vi "Thermal_Camera_Stream.vi"() -> ()   [LabVIEW 2024]
uses:
  <vilib>/userDefined/High Color/IMAQdx.ctl
  <vilib>/vision/driver/NI_Vision_Acquisition_Software.lvlib
panel:
  out "Error Config":errorcluster
  out "error Open":errorcluster
  in  "save":bool
  out "FocusPos":u32
  in  "Scale":u32=13
  in  "Focus >":bool
  in  "Focus <":bool
  in  "Focus":bool
  in  "Numeric":u16
  in  "path":string
  out "error out":errorcluster
  in  "Stop":bool
  in  "Session In":T1="cam4"
  out "Image":T2(plugin-control)
  out "Intensity Graph 2":dbl[][](graph)
  out "Temperature":dbl
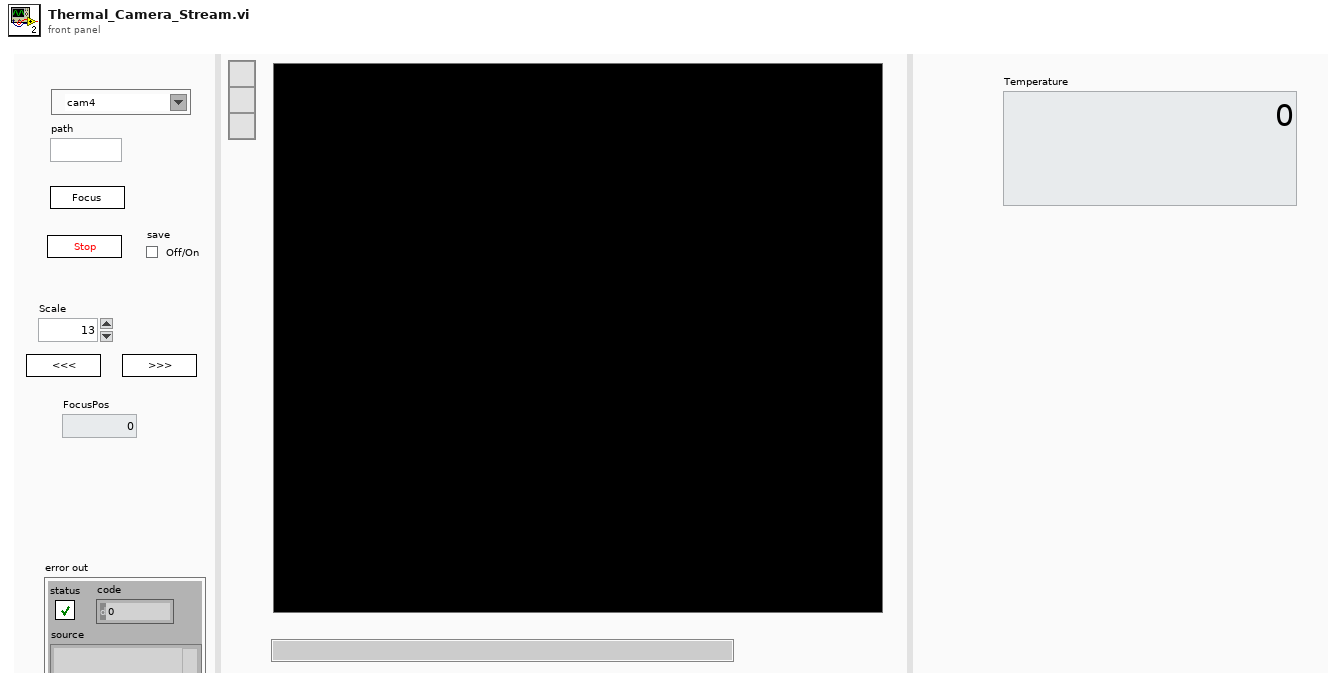
[diagram p1: front panel]
types:
  T1 = typedef "IMAQdx.ctl" = refnum<k21>
  T2 = typedef "IMAQ Image.ctl" = refnum<image>
  T3 = typedef "Image Type" = u32
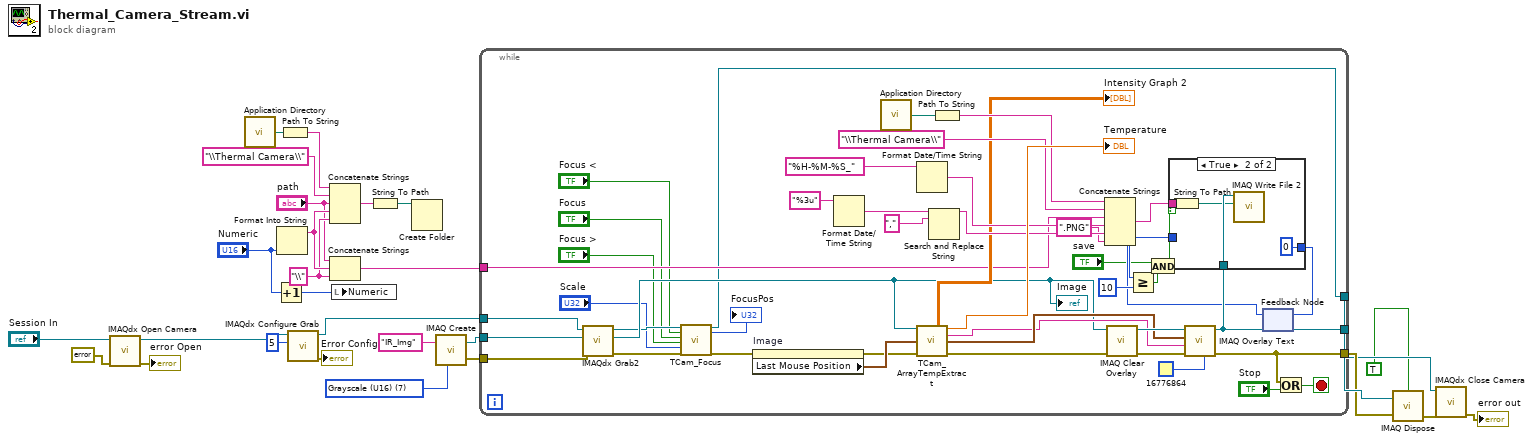
[diagram p0: block diagram]
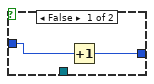
[diagram p2: hidden frame]
diagram:
  w6 = "\\" ("string")
  w17 = T3 7 items=["Grayscale (U8)", "Grayscale (I16)", "Grayscale (SGL)", "Complex (CSG)", "RGB (U32)", "HSL (U32)", "RGB (U64)", "Grayscale (U16)"] ("Image Type")
  n1 = call <vilib>:"IMAQdx Open Camera.vi"("error in"=errorcluster {"status"=FALSE, "code"=0, "source"=""}, "Session In"="Session In") -> ("error out"=→"error Open":errorcluster, "Session Out"=w28:T1)  [unwired: 8 in]
  n2 = call <vilib>:"Application Directory.vi"() -> ("Application Directory"=w16:path)
  n3 = Increment(x="Numeric") -> (x+1=w11:u16)
  n4 = Format Into String("Numeric") -> (resulting string=w7:string)  [unwired: 3 in, 1 out]
  n5 = Path To String(path=w16) -> (string=w14:string)
  n6 = call <vilib>:"IMAQdx Configure Grab.vi"("Number of Buffers"=u32 5, "Session In"=w28) -> ("error out"=→"Error Config":errorcluster, "Session Out"=w26:T1)  [unwired: 8 in]
  n7 = Concatenate Strings(w14, "\\Thermal Camera\\", "path", w7, w6) -> (w13:string)
  n8 = Concatenate Strings("path", w7, w6) -> (w4:string)
  n9 = local write "Numeric"(w11) -> ()
  n10 = String To Path(string=w13) -> (path=w12:path)
  n11 = Create Folder(path (use dialog)=w12) -> ()  [unwired: 2 in, 3 out]
  n12 = call "IMAQ Create"("Image Name"="IR_Img", "Image Type"=w17) -> ("New Image"=w9:T2, "error out"=w8:errorcluster)  [unwired: 3 in]
  n13 = while {
    tunnel: w26 -> [w71]
    tunnel: w8 -> [w70]
    tunnel: [w59] -> w25
    tunnel: [w66] -> w24
    tunnel: [w32] -> w22
    tunnel: w9 -> [w42]
    tunnel: w4 -> [w41]
    stop <- w72 stop-if-true
    n14 = call <vilib>:"IMAQdx Grab2.vi"("error in"=w70, "Image In"=w42, "Session In"=w71) -> ("error out"=w38:errorcluster, "Image Out"=w40:T2, "Session Out"=w39:T1)  [unwired: 5 in, 1 out]
    "Image" <- w40
    n15 = call "TCam_Focus.vi"("Session in"=w39, "Focus <"="Focus <", "Autofocus"="Focus", "Focus >"="Focus >", "Scale"="Scale", "error in (no error)"=w38) -> ("Session Out"=w32:T1, "FocusPos"=→"FocusPos":u32, "error out"=w33:errorcluster)  [unwired: 11 in]
    n16 = property on="Image" class="ImageControl"(error in=w33) -> (error out=w62:errorcluster, "Last Mouse Position"=w63:cluster{"X":i32, "Y":i32})  [unwired: 1 in, 1 out]
    n17 = Format Date/Time String(time format string (%c)="%3u") -> (date/time string=w57:string)  [unwired: 2 in]
    n18 = call <vilib>:"Application Directory.vi"() -> ("Application Directory"=w52:path)
    n19 = Format Date/Time String(time format string (%c)="%H-%M-%S_") -> (date/time string=w56:string)  [unwired: 2 in]
    n20 = call "TCam_ArrayTempExtract.vi"("img in"=w40, "Mouse pos"=w63, "error in (no error)"=w62) -> ("Intensity Graph 4"=→"Intensity Graph 2":dbl[][], "temp"=→"Temperature":dbl, "temp str"=w60:string, "Mouse pos dup"=w61:cluster{"X":i32, "Y":i32}, "error out"=w64:errorcluster)  [unwired: 8 in]
    n21 = Search and Replace String(input string=w57, search string=",") -> (result string=w58:string)  [unwired: 6 in, 3 out]
    n22 = Path To String(path=w52) -> (string=w50:string)
    n23 = Concatenate Strings(w50, "\\Thermal Camera\\", w41, w56, w58, ".PNG" ("string")) -> (w48:string)
    n24 = call "IMAQ Clear Overlay"("error in (no error)"=w64, "Image"=w40) -> ("error out"=w67:errorcluster, "Image Out"=w68:T2)  [unwired: 8 in]
    n25 = call "IMAQ Overlay Text"("BG Color (Transparent)"=u32 16776864, "error in (no error)"=w67, "String"=w60, "Origin"=w61, "Image"=w68) -> ("error out"=w66:errorcluster, "Image Out"=w59:T2)  [unwired: 5 in]
    n26 = feedback #1() -> (w44:u16)  [unwired: 1 in]
    n27 = Greater Or Equal?(x=w44, y=u16 10) -> (x >= y?=w47:bool)
    n28 = And(x="save", y=w47) -> (x .and. y?=w30:bool)
    n29 = case shown="True" w30 {
      tunnel: w59 -> [_ w79]
      tunnel: w48 -> [_ w78]
      tunnel: [w74 u16 0 ("y")] -> w45
      tunnel: w44 -> [w75 _]
      frame False {
        n30 = Increment(x=w75) -> (x+1=w74:u16)
      }
      frame True {
        n31 = String To Path(string=w78) -> (path=w77:path)
        n32 = call-poly "IMAQ Write File 2"("File Path"=w77, "Image"=w79) -> ()  [unwired: 8 in, 2 out]
      }
    }
    n33 = feedback-in #1(w45) -> ()
    n34 = Or(x=w66, y="Stop") -> (x .or. y?=w72:bool)
  }
  n35 = call "IMAQ Dispose"("All Images? (No)"=TRUE, "Image"=w25, "error in (no error)"=w24) -> ("error out"=w23:errorcluster)  [unwired: 3 in]
  n36 = call <vilib>:"IMAQdx Close Camera.vi"("error in"=w23, "Session In"=w22) -> ("error out"=→"error out":errorcluster)  [unwired: 9 in]
